vi "GEOM_GetSelectedAmps.vi"(9 "amplifiers":T1[](array[typedef]) {"fliped" items=["none", "horizontal", "vertical"]; "type" items=["LL", "LR", "UL", "UR"]}, 10 "amplifier in":T1={"number"=0, "type"=0, "rotated"=0, "fliped"=0, "FPAcoord"={"xstart"=1, "ystart"=1}, "Physical_size"={"columns"=0, "rows"=0}, "predata"={"columns"=0, "rows"=0}, "postdata"={"columns"=0, "rows"=0}, "Req ROIs"=[], "Corr ROI"=[], "Detnumber"=0, "ampID"="", "discard"=0} {"fliped" items=["none", "horizontal", "vertical"]; "type" items=["LL", "LR", "UL", "UR"]}) -> (1 "selected amplifiers":T1[](array[typedef]) {"fliped" items=["none", "horizontal", "vertical"]; "type" items=["LL", "LR", "UL", "UR"]})   [LabVIEW 2016]
uses:
  GEOM_Amplifier.ctl
  GEOM_AmpType.ctl
  GEOM_ROI.ctl
  GEOM_Coords.ctl
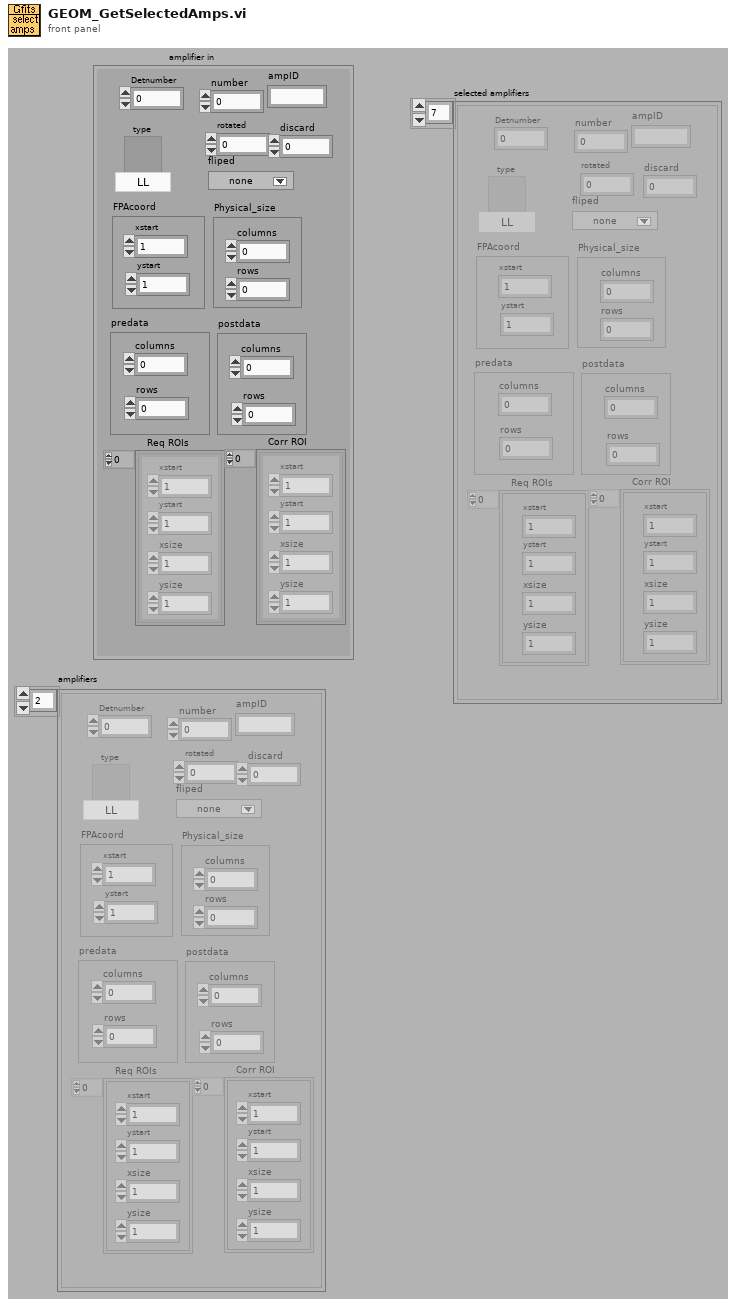
[diagram p1: front panel]
types:
  T1 = typedef "GEOM_Amplifier.ctl" = cluster{"number":i32, "type":T2, "rotated":i16, "fliped":u16, "FPAcoord":cluster{"xstart":i32, "ystart":i32}, "Physical_size":cluster{"columns":i32, "rows":i32}, "predata":cluster{"columns":i32, "rows":i32}, "postdata":cluster{"columns":i32, "rows":i32}, "Req ROIs":T3, "Corr ROI":T3, "Detnumber":i32, "ampID":string, "discard":i32}
  T2 = typedef "GEOM_AmpType.ctl" = u16
  T3 = typedef "GEOM_ROI.ctl" = T4[]
  T4 = typedef "GEOM_Coords.ctl" = cluster{"xstart":u32, "ystart":u32, "xsize":u32, "ysize":u32}
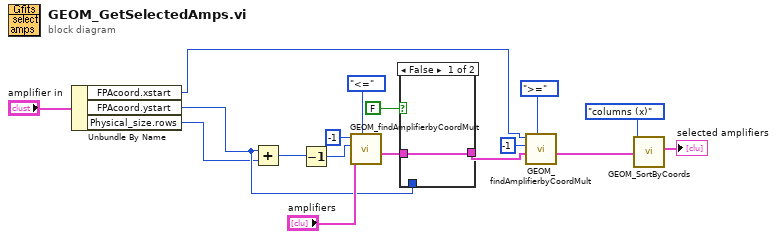
[diagram p0: block diagram]
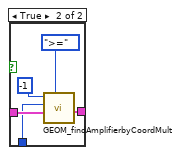
[diagram p2: hidden frame]
diagram:
  n1 = Unbundle By Name("amplifier in") -> ("FPAcoord.xstart"=w5:i32, "FPAcoord.ystart"=w3:i32, "Physical_size.rows"=w2:i32)
  n2 = Add(x=w3, y=w2) -> (x+y=w17:i32)
  n3 = Decrement(x=w17) -> (x-1=w7:i32)
  n4 = call "GEOM_findAmplifierbyCoordMult.vi"("mode"=enum16{"=", "<", ">", "<=", ">="}."<=", "amplifiers"="amplifiers", "ycoord"=w7, "xcoord"=-1) -> ("amplifiers"=w14:T1[])  [unwired: 7 out]
  n5 = case shown="False" FALSE {
    tunnel: w14 -> [w18 w21]
    tunnel: [w18 w20] -> w1
    tunnel: w3 -> [_ w19]
    frame False {
    }
    frame True {
      n6 = call "GEOM_findAmplifierbyCoordMult.vi"("mode"=enum16{"=", "<", ">", "<=", ">="}.">=", "amplifiers"=w21, "ycoord"=w19, "xcoord"=-1) -> ("amplifiers"=w20:T1[])  [unwired: 7 out]
    }
  }
  n7 = call "GEOM_findAmplifierbyCoordMult.vi"("mode"=enum16{"=", "<", ">", "<=", ">="}.">=", "amplifiers"=w1, "ycoord"=-1, "xcoord"=w5) -> ("amplifiers"=w10:T1[])  [unwired: 7 out]
  n8 = call "GEOM_SortByCoords.vi"("amplifiers"=w10, "how"=enum16{"rows (y)", "columns (x)"}."columns (x)") -> ("sorted amplifiers"=→"selected amplifiers":T1[])  [unwired: 9 out]
